vi "niFPGA FFT Twiddle Symmetry.vi"(0 "twiddle index":u16, 12 "N/4":u16) -> (4 "modified twiddle index":u16, 14 "flag":fxp<+,2,2>)   [LabVIEW 2017]
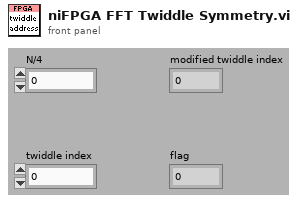
[diagram p1: front panel]
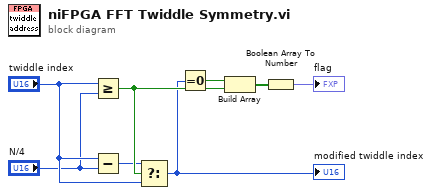
[diagram p0: block diagram]
diagram:
  n1 = Greater Or Equal?(x="twiddle index", y="N/4") -> (x >= y?=w6:bool)
  n2 = Subtract(x="twiddle index", y="N/4") -> (x-y=w3:u16)
  n3 = Select(t=w3, s=w6, f="twiddle index") -> (s? t:f=w2:u16)
  "modified twiddle index" <- w2
  n4 = Equal To 0?(x=w2) -> (x = 0?=w7:bool)
  n5 = Build Array(w7, w6) -> (w8:bool[])
  n6 = Boolean Array To Number(Boolean array=w8) -> (number=→"flag":fxp<+,2,2>)
